vi "part3.vi"() -> ()   [LabVIEW 2019]
panel:
  out "GRE":bool
  out "YEL":bool
  out "RED":bool
  in  "stop":bool
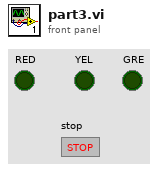
[diagram p1: front panel]
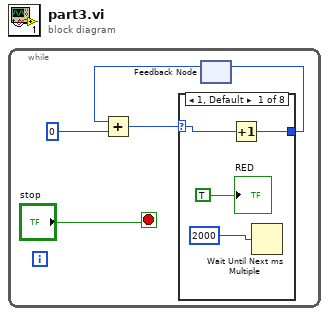
[diagram p0: block diagram]
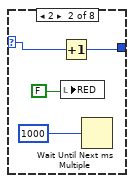
[diagram p2: hidden frame]
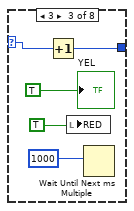
[diagram p3: hidden frame]
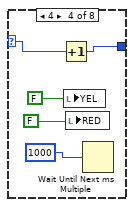
[diagram p4: hidden frame]
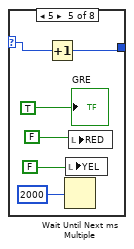
[diagram p5: hidden frame]
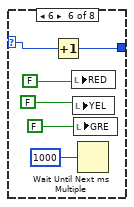
[diagram p6: hidden frame]
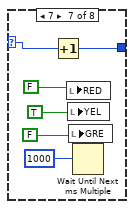
[diagram p7: hidden frame]
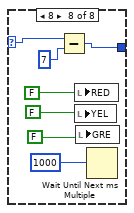
[diagram p8: hidden frame]
diagram:
  n1 = while {
    stop <- "stop" stop-if-true
    n2 = feedback #1() -> (w3:i32)  [unwired: 1 in]
    n3 = Add(x=w3, y=0) -> (x+y=w5:i32)
    n4 = case shown="1, Default" w5 {
      selector: w5 -> [w8 w12 w16 w21 w26 w32 w38 w45]
      tunnel: [w7 w11 w15 w20 w25 w31 w37 w43] -> w4
      frame 1, Default {
        n5 = Increment(x=w8) -> (x+1=w7:i32)
        n6 = Wait Until Next ms Multiple(millisecond multiple=2000) -> ()  [unwired: 1 out]
        "RED" <- TRUE
      }
      frame 2 {
        n7 = Increment(x=w12) -> (x+1=w11:i32)
        n8 = local write "RED"(FALSE) -> ()
        n9 = Wait Until Next ms Multiple(millisecond multiple=1000) -> ()  [unwired: 1 out]
      }
      frame 3 {
        n10 = Increment(x=w16) -> (x+1=w15:i32)
        n11 = local write "RED"(TRUE) -> ()
        n12 = Wait Until Next ms Multiple(millisecond multiple=1000) -> ()  [unwired: 1 out]
        "YEL" <- TRUE
      }
      frame 4 {
        n13 = Increment(x=w21) -> (x+1=w20:i32)
        n14 = local write "YEL"(FALSE) -> ()
        n15 = local write "RED"(FALSE) -> ()
        n16 = Wait Until Next ms Multiple(millisecond multiple=1000) -> ()  [unwired: 1 out]
      }
      frame 5 {
        n17 = Increment(x=w26) -> (x+1=w25:i32)
        n18 = Wait Until Next ms Multiple(millisecond multiple=2000) -> ()  [unwired: 1 out]
        n19 = local write "YEL"(FALSE) -> ()
        n20 = local write "RED"(FALSE) -> ()
        "GRE" <- TRUE
      }
      frame 6 {
        n21 = Increment(x=w32) -> (x+1=w31:i32)
        n22 = local write "RED"(FALSE) -> ()
        n23 = local write "YEL"(FALSE) -> ()
        n24 = local write "GRE"(FALSE) -> ()
        n25 = Wait Until Next ms Multiple(millisecond multiple=1000) -> ()  [unwired: 1 out]
      }
      frame 7 {
        n26 = Increment(x=w38) -> (x+1=w37:i32)
        n27 = local write "RED"(FALSE) -> ()
        n28 = local write "YEL"(TRUE) -> ()
        n29 = local write "GRE"(FALSE) -> ()
        n30 = Wait Until Next ms Multiple(millisecond multiple=1000) -> ()  [unwired: 1 out]
      }
      frame 8 {
        n31 = Subtract(x=w45, y=7) -> (x-y=w43:i32)
        n32 = local write "RED"(FALSE) -> ()
        n33 = local write "YEL"(FALSE) -> ()
        n34 = local write "GRE"(FALSE) -> ()
        n35 = Wait Until Next ms Multiple(millisecond multiple=1000) -> ()  [unwired: 1 out]
      }
    }
    n36 = feedback-in #1(w4) -> ()
  }
